vi "Write Sync Line.vi"(8 "error in (no error)":errorcluster, 10 "Sync Line":tag, 11 "Synchronization Device in":refnum<class "Synchronization Device.lvclass">) -> (0 "error out":errorcluster, 3 "Synchronization Device out":refnum<class "Synchronization Device.lvclass">)   [LabVIEW 2018]
uses:
  Synchronization Device.lvclass
  C:/LVCUR/flash-gordon/Hardware/Device/Device.lvclass
  C:/Program Files/National Instruments/LabVIEW 2018/vi.lib/ActorFramework/Actor/Actor.lvclass
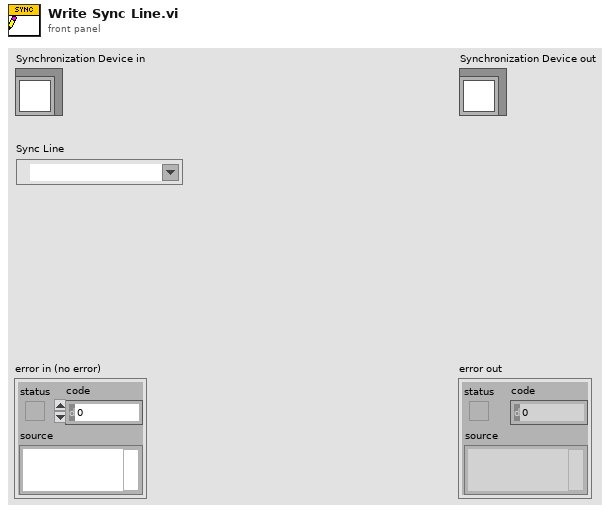
[diagram p1: front panel]
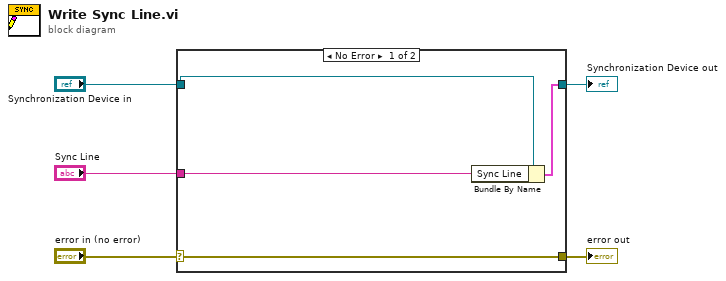
[diagram p0: block diagram]
diagram:
  n1 = case shown="No Error" "error in (no error)" {
    selector: "error in (no error)" -> [w9 w10]
    tunnel: [w9 w10] -> w4
    tunnel: [w7 w11] -> w2
    tunnel: "Synchronization Device in" -> [w8 w11]
    tunnel: "Sync Line" -> [w6 _]
    frame No Error {
      n2 = Bundle By Name(cluster=w8, "Sync Line"=w6) -> (w7:cluster{})
    }
    frame Error {
    }
  }
  "error out" <- w4
  "Synchronization Device out" <- w2
